vi "Configure Burst.vi"(0 "VISA resource name":refnum<visa-resource-name>, 1 "Enable Burst (T: Enable)":bool=TRUE, 2 "Burst Phase Angle (0 Degree)":dbl, 5 "Channel (1: 1)":i32(ring)=1 items=["1"=1, "2"=2], 7 "Burst Mode (0: Triggered)":i32(ring) items=["Triggered", "Gated"], 9 "Burst Gate Polarity (0: Normal)":i32(ring) items=["Normal", "Inverted"], 11 "error in (no error)":errorcluster, 12 "Infinite Cycle (T: Enable)":bool=TRUE, 13 "Cycle Count (1)":i32(ring)=1 items=["1"=1, "2"=2], 14 "Burst Internal Period (10 ms)":dbl=10.0) -> (4 "VISA resource name out":refnum<visa-resource-name>, 15 "error out":errorcluster)   [LabVIEW 2013, in "AWG.lvlib" / "Agilent 3352X Series.lvlib"]
doc: "Allows and configures burst. Configures the function generator to output a waveform with specified number of cycles, called burst. The carrier waveform shape and parameters are set by Configure Standard Waveform.\n\n<b>Note</b>:\n(1) Before using this mode, all other modes must be turned off."
uses:
  Agilent 3352X Series.lvlib
panel:
  # "Triggered BM Settings"
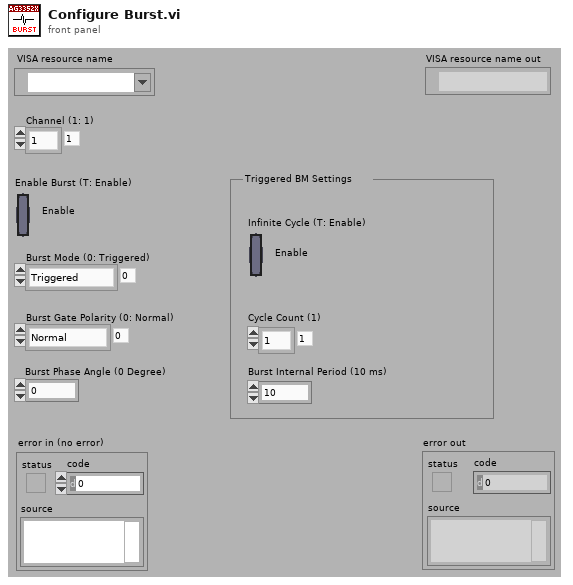
[diagram p1: front panel]
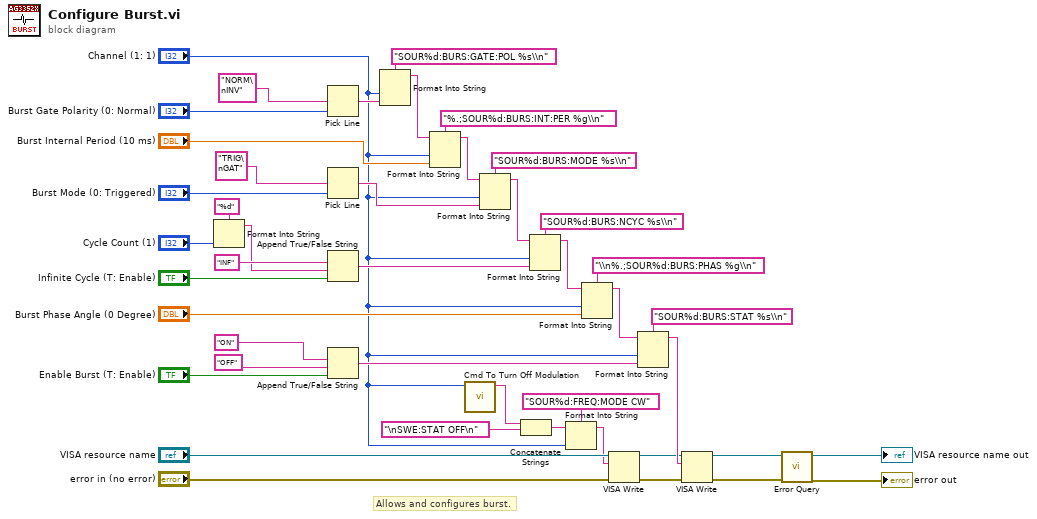
[diagram p0: block diagram]
diagram:
  # "Allows and configures burst."
  n1 = Format Into String(format string="%d", "Cycle Count (1)") -> (resulting string=w14:string)  [unwired: 2 in, 1 out]
  n2 = Pick Line(multi-line string="NORM\nINV", line index="Burst Gate Polarity (0: Normal)") -> (output string=w17:string)  [unwired: 1 out]
  n3 = Pick Line(multi-line string="TRIG\nGAT", line index="Burst Mode (0: Triggered)") -> (output string=w36:string)  [unwired: 1 out]
  n4 = Append True/False String(1:"Infinite Cycle (T: Enable)", 2:w14, 3:"INF") -> (0:w22:string)  [unwired: 1 out]
  n5 = Append True/False String(1:"Enable Burst (T: Enable)", 2:"OFF", 3:"ON") -> (0:w28:string)  [unwired: 1 out]
  n6 = Format Into String(format string="SOUR%d:BURS:GATE:POL %s\\n", "Channel (1: 1)", w17) -> (resulting string=w43:string)  [unwired: 2 in, 1 out]
  n7 = Format Into String(format string="%.;SOUR%d:BURS:INT:PER %g\\n", initial string=w43, "Channel (1: 1)", "Burst Internal Period (10 ms)") -> (resulting string=w38:string)  [unwired: 1 in, 1 out]
  n8 = call "Cmd To Turn Off Modulation.vi"("Channel (1: 1)"="Channel (1: 1)") -> ("Cmd String"=w5:string)  [unwired: 10 out]
  n9 = Format Into String(format string="SOUR%d:BURS:MODE %s\\n", initial string=w38, "Channel (1: 1)", w36) -> (resulting string=w35:string)  [unwired: 1 in, 1 out]
  n10 = Concatenate Strings(w5, "\nSWE:STAT OFF\n") -> (w3:string)
  n11 = Format Into String(format string="SOUR%d:BURS:NCYC %s\\n", initial string=w35, "Channel (1: 1)", w22) -> (resulting string=w13:string)  [unwired: 1 in, 1 out]
  n12 = Format Into String(format string="SOUR%d:FREQ:MODE CW", initial string=w3, "Channel (1: 1)") -> (resulting string=w2:string)  [unwired: 1 in, 1 out]
  n13 = Format Into String(format string="\\n%.;SOUR%d:BURS:PHAS %g\\n", initial string=w13, "Channel (1: 1)", "Burst Phase Angle (0 Degree)") -> (resulting string=w21:string)  [unwired: 1 in, 1 out]
  n14 = VISA Write(VISA resource name="VISA resource name", write buffer=w2, error in (no error)="error in (no error)") -> (VISA resource name out=w8:refnum<visa-resource-name>, error out=w7:errorcluster)  [unwired: 1 out]
  n15 = Format Into String(format string="SOUR%d:BURS:STAT %s\\n", initial string=w21, "Channel (1: 1)", w28) -> (resulting string=w20:string)  [unwired: 1 in, 1 out]
  n16 = VISA Write(VISA resource name=w8, write buffer=w20, error in (no error)=w7) -> (VISA resource name out=w27:refnum<visa-resource-name>, error out=w26:errorcluster)  [unwired: 1 out]
  n17 = call "Error Query.vi"("error in (no error)"=w26, "VISA resource name"=w27) -> ("error out"=→"error out":errorcluster, "VISA resource name out"=→"VISA resource name out":refnum<visa-resource-name>)  [unwired: 8 out]
